vi "Send Update Controller State.vi"(7 "Message Priority (Normal)":T2=enum."Normal", 8 "error in (no error)":errorcluster, 10 "Car Wash Controller State":T1, 11 "Message Enqueuer":refnum<class "Message Enqueuer.lvclass">) -> (0 "error out":errorcluster, 3 "Message Enqueuer out":refnum<class "Message Enqueuer.lvclass">)   [LabVIEW 2012, in "Car Wash Controller.lvlib" / "Update Controller State Msg.lvclass"]
doc: "This VI sends the message to an actor."
uses:
  Update Controller State Msg.lvclass
  <vilib>/ActorFramework/Message Enqueuer/Message Enqueuer.lvclass
  <vilib>/ActorFramework/Message Enqueuer/Message Priority.ctl
  Car Wash Controller/Car Wash Controller State.ctl
  Update Controller State Msg.lvclass/Update Controller State Msg.ctl
  <vilib>/ActorFramework/Message Enqueuer/Message Enqueuer.lvclass/Message Enqueuer.ctl
  <vilib>/ActorFramework/Message Priority Queue/Priority Enqueue.vi
  Car Wash Controller/Car Wash Controller.lvclass
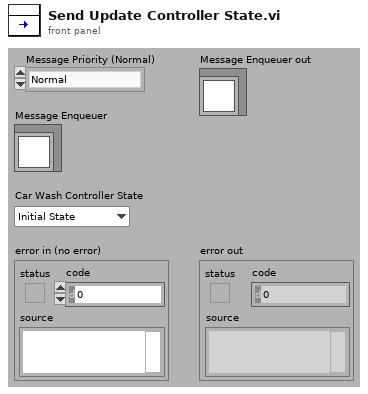
[diagram p1: front panel]
types:
  T1 = typedef "Car Wash Controller.lvlib/Car Wash Controller.lvclass/Car Wash Controller State.ctl" = enum16{"Initial State", "Wait For Start State", "Start State", "Wait For Vehicle Position State", "Wash Step Execution State", "Wash Step / Cycle Completion State", "Wash Exit State", "Wash Abort / Terminate State"}
  T2 = typedef "Actor Framework.lvlib/Message Enqueuer.lvclass/Message Priority.ctl" = enum16{"Low", "Normal", "High"}
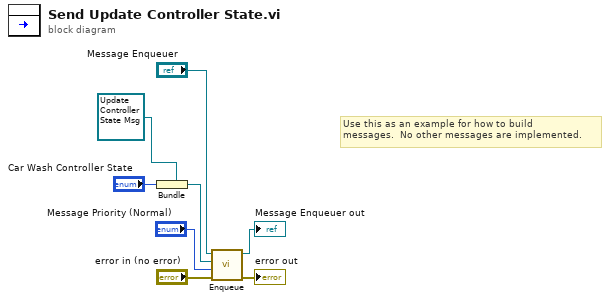
[diagram p0: block diagram]
diagram:
  # "Use this as an example for how to build\nmessages.  No other messages are implemented."
  n1 = Bundle(cluster=refnum<class "Update Controller State Msg.lvclass"> refnum ("Object"), "Car Wash Controller State") -> (w4:refnum<class "Update Controller State Msg.lvclass">)
  n2 = call <vilib>:"Enqueue.vi"("error in (no error)"="error in (no error)", "Message Priority (Normal)"="Message Priority (Normal)", "Message"=w4, "Message Enqueuer in"="Message Enqueuer") -> ("error out"=→"error out":errorcluster, "Message Enqueuer out"=→"Message Enqueuer out":refnum<class "Message Enqueuer.lvclass">)  [unwired: 6 in]
